vi "HitrapGUI.contents.vi"   [LabVIEW 2014, in "HitrapGUI.lvlib"]
uses:
  HitrapGUI.lvlib
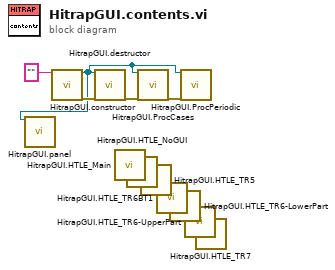
[diagram p0: block diagram]
diagram:
  n1 = call "HitrapGUI.constructor.vi"("name"="") -> ("i ref out"=w1:refnum<vi>, "error out"=w5:errorcluster)  [unwired: 16 in, 1 out]
  n2 = call "HitrapGUI.panel.vi"("object ref"=w1) -> ()  [unwired: 18 in, 1 out]
  n3 = call "HitrapGUI.destructor.vi"("i ref in"=w1, "error in (no error)"=w5) -> ("error out"=w4:errorcluster)  [unwired: 17 in]
  n4 = call "HitrapGUI.HTLE_Main.vi"() -> ()  [unwired: 1 in]
  n5 = call "HitrapGUI.HTLE_NoGUI.vi"() -> ()  [unwired: 1 in]
  n6 = call "HitrapGUI.ProcCases.vi"("i ref in"=w1, "error in (no error)"=w4) -> ("error out"=w3:errorcluster)  [unwired: 15 in, 2 out]
  n7 = call "HitrapGUI.HTLE_TR5.vi"() -> ()  [unwired: 1 in]
  n8 = call "HitrapGUI.HTLE_TR6BT1.vi"() -> ()  [unwired: 1 in]
  n9 = call "HitrapGUI.HTLE_TR6-LowerPart.vi"() -> ()  [unwired: 1 in]
  n10 = call "HitrapGUI.ProcPeriodic.vi"("i ref in"=w1, "error in (no error)"=w3) -> ()  [unwired: 15 in, 3 out]
  n11 = call "HitrapGUI.HTLE_TR6-UpperPart.vi"() -> ()  [unwired: 1 in]
  n12 = call "HitrapGUI.HTLE_TR7.vi"() -> ()  [unwired: 1 in]
